vi "Keyence.Gui.vi"(8 "error in":errorcluster, 11 "Idx":i32) -> (0 "error out":errorcluster)   [LabVIEW 2016]
doc: "The function checks for actual position and move to desired absolute position. Then depending on the settings function can check again for position and make retries with lower speed.\n\n#retries - the number of retries to move the motor exactly to position; each time new move is done the speed is divided by 4 (but the min speed is 1) in order to move precisely to positon. possible values are:\n-1: only movement is done without checking whether position was reached\n0: one movemnt is done and then checking whether position was reached\n1: the max number of retries after one unsuccessful movents; with each new movment speed is decreased by 4 and new check is done; if the posiition is in given range function is done\n\nrange[mm] - the max range when checking for the position in range; the minimal value is 0.01mm; the position status is returned as \"Status\" flags"
uses:
  Keyence.BankGui1.ctl
  Keyence.BankGui2.ctl
  Keyence.Data.Status.State.ctl
  Station/Station.State.ctl
  tools/Translator/Translator.Message.ctl
  tools/Translator/Translator.FormatMessage.vi
  Global/ApplicationGlobal.vi
  tools/Config/Config.Global.vi
  Keyence.Global.vi
  Station/Station.Global.vi
  tools/Translator/Translator.Global.vi
panel:
  in  "AutoTune":bool
  in  "Bank2":T1 caption="Bank"
  out "Status":string caption="Code 2"
  out "CodeLevel":string
  out "CodeClass":string
  out "Code":string
  in  "ExitButton":bool
  out "Hider":bool
  in  "ResetPeriod":i32 caption="Reset [s]"
  in  "ReconenctPeriod":i32 caption="Reconect [s]"
  in  "Bank":T2
  in  "Timeout [ms]":i32=1000
  in  "Retries":i32
  in  "IP":string="192.168.0.10"
  out "Image":picture
  out "Hider2":bool
  in  "ScanButton":bool
  in  "TuneButton":bool
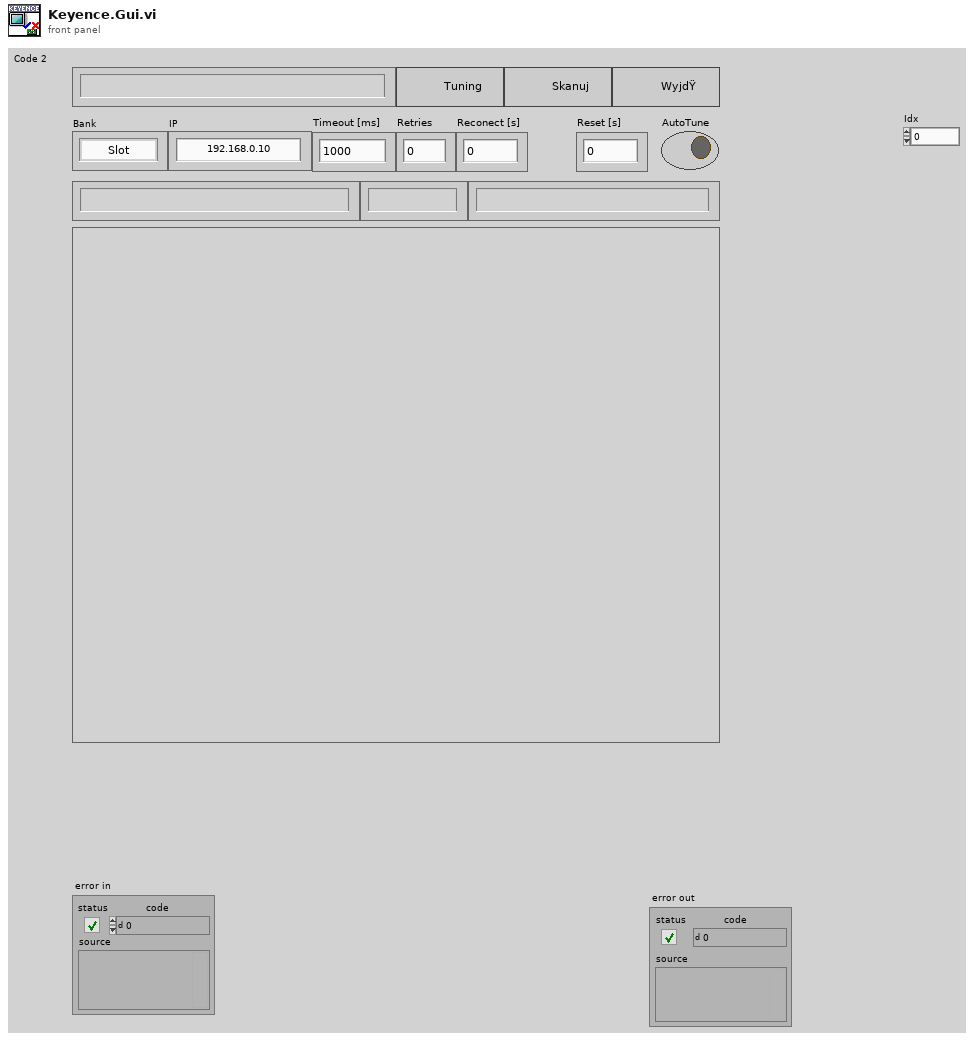
[diagram p1: front panel]
types:
  T1 = typedef "Keyence.BankGui2.ctl" = enum8{"WabcoProd", "WabcoPlate", "ClientProd", "ClientPlate", "TotalQuant", "SerialNo"}
  T2 = typedef "Keyence.BankGui1.ctl" = enum8{"Slot", "A-1", "B-1", "A-2", "B-2"}
  T3 = enum8{"Enabled", "Disabled", "Disabled and Grayed Out"}
  T4 = typedef "Station.State.ctl" = enum16{"Idle", "Ready", "Run", "Stop", "Error", "Home", "Done", "Emg"}
  T5 = typedef "Keyence.Data.Status.State.ctl" = enum16{"First", "Init", "Reset", "Idle", "Scan", "Tune"}
  T6 = typedef "Translator.Message.ctl" = enum16{"-", "Event confirmed", "Log out", "Log in", "Shutdown", "Cancel", "Start", "Begin time", "End time", "Duration", "Service Mode", "Ignore Results", "Serial Format", "On", "Off", "OK", "NOK", "NOK %s", "Home", "Work", "Close", "Open", "In progress...", "Missing", "Empty", "Hardware failure", "Initial", "Default", "Total", "Out of range", "Free disk space is below 1GB - contact technician", "Error %d >> %s", "Error %d >> %s >> %s", "Msg %d >> %s", "Laser msg %d %s", "Laser cmd error %s %d", "Laser cmd failed %s", "Laser cmd warning %s", "Laser disconnected", "Laser status %s", "Laser already started", "Laser job unkonwn %s", "Laser job missing %s", "Laser job select failure %s", "Unable to start laser printing (%s)", "Unable to stop laser printing (%s)", "Laser marking aborted", "Laser marking timeout", "Unable to reset Laser Interlock (%s)", "Unable to trigger Laser. Laser not ready (%s)", "Laser job '%s' coordinates not configured", "Starting %s", "Quitting %s", "Configured", "Initializing", "Quitting", "Loading", "Loaded %d results", "Loaded %d events", "Running", "Stopped", "Summary", "Laser", "Do you want to continue?", "Do you want to delete the configuration?", "The configuration is being used by an order. Unable to delete!", "Press confirm button", "Station is not based. Do you want to exit?", "Station requires changeover. Do you want to run the test?", "Test options are not set as default. Do you want to continue?", "Formatting of WabcoNo is disabled. Do you want to continue?", "Product not detected. Do you want to continue?", "Product scan failed. Do you want to continue?", "Calibration", "Log out?", "System", "All", "IDLE", "Translating...%s", "Not found", "Alarm %s", "Run", "Skip", "Abort", "Repeat", "Please wait...", "Database disconnected", "Database disconnected - changeover disabled!", "Login to database successful", "Login to database failed: %d; %s", "Unable to check the product status of reference %d - database disconnected", "Unable to set the product status of reference %d - database disconnected", "Variant file backup %s", "Read variant (%s)", "Result", "Station armed!", "Station requires changeover!", "Select reference number...", "EMERGENCY BUTTON - press Control button", "EMERGENCY DOOR - press Control button", "Resetting Emergency...", "Unable to reset safety circuit - Emergency Button pressed", "Unable to reset safety circuit - Emergency Side Door open", "Station not based", "Station based", "Station not empty", "Station basing...", "No order", "Press Start to begin new order", "Scanning new order", "Order NOK. Correct or scan again", "Order OK. Press Accept", "Order ready", "Revolver incorrect", "Fork incorrect", "Revolver missing", "Revolver empty", "Container missing", "Offline results", "Offline statistics", "Updating statistics %.1f %%", "DMC Configurator", "Door open", "Close the front door", "Press start button", "Done. Open the front door", "Running...", "Running...%.1f %%", "Pause %s", "Pause %s. NOK container missing", "Pause %s. OK container missing", "Pause %s. Revolver empty", "Pause %s. Revolver missing", "Pause %s. Revolver incorrect", "Pause %s. Fork missing", "Pause %s. Fork incorrect", "Pause %s. Too many failures", "Pause %s. Unloading failure", "Pause %s. One slot is not working", "Pause %s. Part order is done. Empty OK container", "Pause %s. Unable to move product to slot", "Pause %s. Unable to move back product pusher", "Pause %s. Unable to lift product", "Pause %s. Unable to move back product lifter", "Pause %s. Unable to move product arm to Work", "Pause %s. Unable to move product arm to NOK", "Pause %s. Unable to move product arm to OK", "Pause %s. Unable to unsuck the NOK product", "Pause %s. Unable to drop the NOK product", "Pause %s. Product OK missing", "Pause %s. Unable to unsuck the OK product", "Pause %s. Unable to drop the OK product", "Stopping...", "File '%s' is missing", "File '%s' is broken", "File '%s' is running", "Log file started (%s)", "Log file ended (%s)", "Log file stopped (%s)", "Log file ignored (%s)", "Log file exported (%s)", "Log file export failed (%s)", "Wrong serial number in log file", "Wrong reference number in log file", "Test steps are missing", "%s = %.3f", "Process param '%s' not found in DB", "Process param '%s' wrong order", "Process param '%s' value %.3f out of limits (%.3f; %.3f)", "Step%d param '%s' not found in DB", "Step%d param '%s' wrong order", "Step%d param '%s' value %.3f out of limits (%.3f; %.3f)", "Step%d EV '%s' not found in DB", "Step%d EV '%s' wrong order", "\"%s\" not found in DB", "\"%s\" wrong order", "\"%s\" value %.3f out of limits (%.3f; %.3f)", "\"%s\" not found in software", "Process init (%s)", "Process started", "Process restarted", "Process run", "Process done", "Process done - remove OK container", "Process aborted", "Process aborted at work", "Process aborted at home", "Process error", "Process error at home", "Process error at work", "Process close", "Process pause", "Process continue", "Process door open", "Process door close", "Process pause at slot %s due to %s", "Select plate from the order to process", "Do you want to start the process?", "Do you want to continue the process?", "There is unfinished order. Do you want to put the new order?", "Product %s %d OK", "Product %s %d NOK", "Unable to unload the slot %s. Product missing in the slot", "Unable to unload the slot %s. Product already in the arm", "Unable to accept the product as OK. Product missing in slot %s", "Unable to accept the product as OK. Product could not drop into the container at slot %s", "Unable to accept the product as NOK. Product could not drop into the container at slot %s", "Scan failed. Error %s", "Scan failed. Scanner disconnected", "Scan failed. Wrong Wabco number %d, limit (%d,%d)", "Scan failed. Wrong serial number %d, limit (%d,%d)", "Scan failed. Wrong date %d, limit (%d,%d)", "Scan failed. Wrong product wabco number %d (expected %d)", "Scan failed. Wrong product serial number %d (expected > 0)", "Scan OK %s", "Scan failed. Unable to determine table position (%s)", "Scan failed. Timeout", "Tune failed. Scanner disconnected", "Tune failed. Timeout", "%s = %d", "%s = %d->%d", "Unable to set %s = %.2f - Air Pressure Inside off", "Unable to set digital output '%s' = %d", "Unable to activate air pressure inside - timeout", "Unable to activate air pressure inside - aborted", "Unable to switch on Air Main Valve - Air Pressure Inlet off", "Unable to switch on Air Main Valve - Door open", "Unable to switch off Air Main Valve - timeout", "Unable to switch off Air Main Valve - aborted", "Unable to rotate Table - timeout", "Unable to rotate Table - aborted", "Unable to rotate Table - Product Move not in Home position", "Unable to rotate Table - Air Pressure Inside off", "Unable to rotate Table - Product Lift A not in Home position", "Unable to rotate Table - Product Lift B not in Home position", "Unable to rotate Table - unlock before movement timeout", "Unable to rotate Table - lock after movement timeout", "Unable to move Table Lock to %s position - timeout", "Unable to move Table Lock to %s position - aborted", "Unable to move Table Lock to %s position - Air Pressure Inside off", "Unable to move Table Lock to %s position - Table not in position", "Unable to move Product Lift A to %s position - timeout", "Unable to move Product Lift B to %s position - timeout", "Unable to move Product Lift A to %s position - aborted", "Unable to move Product Lift B to %s position - aborted", "Unable to move Product Lift A to %s position - Air Pressure Inside off", "Unable to move Product Lift B to %s position - Air Pressure Inside off", "Unable to move Product Lift A to %s position - Table not locked", "Unable to move Product Lift B to %s position - Table not locked", "Unable to move Product Lift A to %s position - Product Arm not in Work position", "Unable to move Product Lift B to %s position - Product Arm not in Work position", "Unable to set Product Suction Gripper %s to %s - timeout", "Unable to set Product Suction Gripper %s to %s - aborted", "Unable to set Product Suction Gripper %s to %s - Air Pressure Inside off", "Unable to set Product Suction Gripper %s to %s - Table slot unkown", "Unable to move Product Arm to %s position - timeout", "Unable to move Product Arm to %s position - aborted", "Unable to move Product Arm to %s position - Air Pressure Inside off", "Unable to move Product Arm to %s position - Product Lift A not in Home position", "Unable to move Product Arm to %s position - Product Lift B not in Home position", "Unable to move Product to %s position - timeout", "Unable to move Product to %s position - aborted", "Unable to move Product to %s position - Air Pressure Inside off", "Unable to move Product to %s position - Table not in position"}
  T7 = typedef "Keyence.Data.Status.ctl" = cluster{"State":T5, "Ref":refnum<k5>, "Bank":u8, "Version":string, "Model":string, "EndTS":timestamp, "ImgPath":path, "Tuned":bool}
  T8 = typedef "Keyence.CodeDetails.ctl" = cluster{"text":string, "status":bool, "corners":cluster{"X":i32, "Y":i32}[], "level":u8, "class":string, "path":path}
  T9 = typedef "Keyence.Data.Sets.ctl" = cluster{"IP":string, "Timeout_ms":i32, "Retries":i32, "ReconnectPeriod_s":i32, "ResetPeriod_s":i32, "ReadImg":bool}
  T10 = typedef "imagedata.ctl" = cluster{"image type":i32, "image depth":i32, "image":u8[], "mask":u8[], "colors":u32[], "Rectangle":cluster{"left":i16, "top":i16, "right":i16, "bottom":i16}}
  T11 = typedef "Station.Data.ctl" = cluster{"State":T4, "Seq.State":T12, "Seq.BreakReason":T13, "Seq.BreakSource":T14, "Hw failure":bool, "Unconfirmed":bool, "Station empty":bool, "Home err":bool, "Order done":bool, "DUT present":T15, "EmgState":T16, "Sets":T17, "StatusBits":T20}
  T12 = typedef "Sequence.State.ctl" = enum16{"Init", "Idle", "Home", "Work", "Run", "Pause"}
  T13 = typedef "Sequence.Test.BreakReason.ctl" = enum16{"-", "NOK container", "OK container", "Rev empty", "Rev missing", "Rev wrong", "Fork missing", "Fork wrong", "NOK limit", "Unload failure", "Single slot", "Part done", "Err: Prod move work", "Err: Prod move home", "Err: Prod lift work", "Err: Prod lift home", "Err: Prod Arm Work", "Err: Prod Arm NOK", "Err: Prod Arm OK", "Err: Prod NOK suck", "Err: Prod NOK drop", "Err: Prod OK missing", "Err: Prod OK suck", "Err: Prod OK drop"}
  T14 = typedef "Sequence.Test.BreakSource.ctl" = enum16{"-", "A", "B", "A/B"}
  T15 = typedef "FestoCPX.Station.ProdPresent.ctl" = cluster{"Slot1":cluster{"A":bool, "B":bool}, "Slot2":cluster{"A":bool, "B":bool}, "Slot3":cluster{"A":bool, "B":bool}, "Slot4":cluster{"A":bool, "B":bool}, "Final":cluster{"A":bool, "B":bool}, "OK":cluster{"A":bool, "B":bool}, "Container":cluster{"OK":bool, "NOK":bool}}
  T16 = typedef "FestoCPX.Station.EmgState.ctl" = cluster{"Button":bool, "SideDoor":bool, "FrontDoor":bool, "DoorSecured":bool}
  T17 = typedef "Sequence.UserData.ctl" = cluster{"GuiMode":T18, "Test":T19, "ContinueOrder":bool}
  T18 = typedef "Sequence.MainMode.ctl" = enum16{"Process", "Base", "Order", "Manual", "Logs", "Results", "Stats", "DMC Config"}
  T19 = typedef "MainGui.TestOptions.ctl" = cluster{"IgnoreResults":bool, "IgnoreImages":bool, "ServiceMode":bool}
  T20 = typedef "Station.Home.Status.Bits.ctl" = cluster{"Door Close":bool, "Rev OK":bool, "Fork OK":bool, "Container OK":bool, "Station empty":bool}
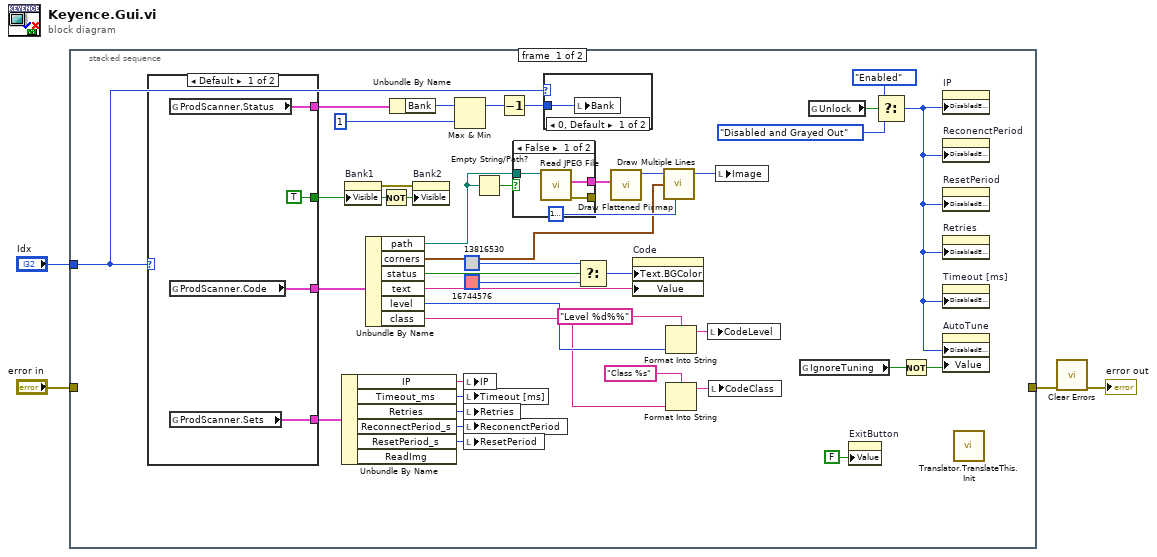
[diagram p0: block diagram]
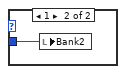
[diagram p2: hidden frame]
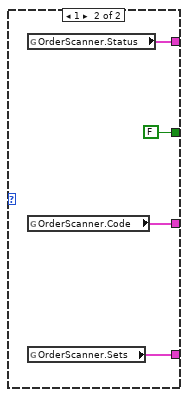
[diagram p3: hidden frame]
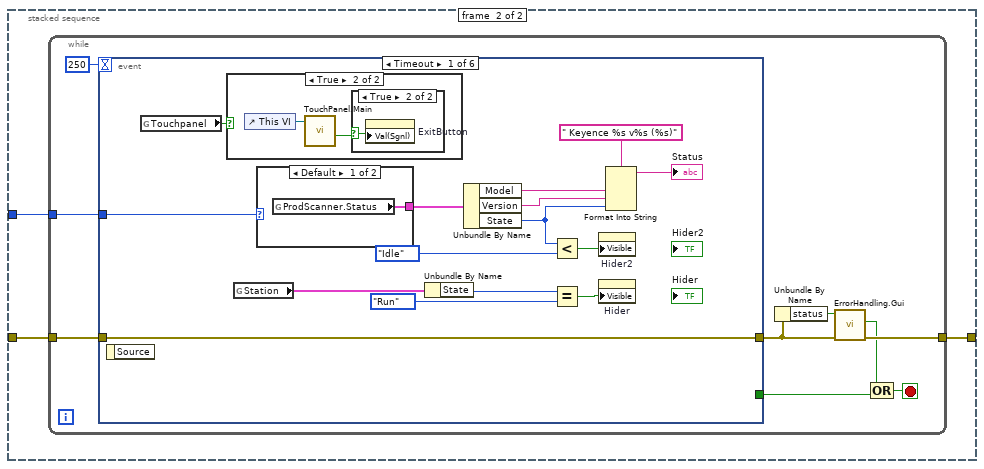
[diagram p5: hidden frame]
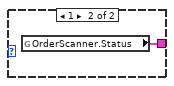
[diagram p6: hidden frame]
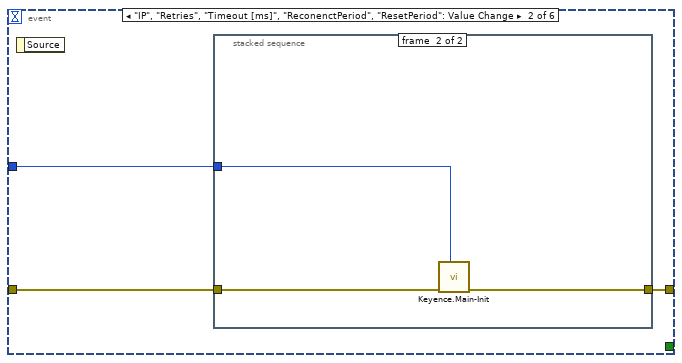
[diagram p9: hidden frame]
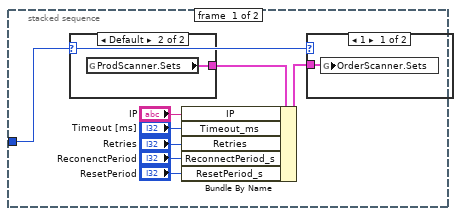
[diagram p10: hidden frame]
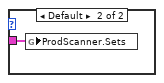
[diagram p11: hidden frame]
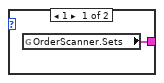
[diagram p12: hidden frame]
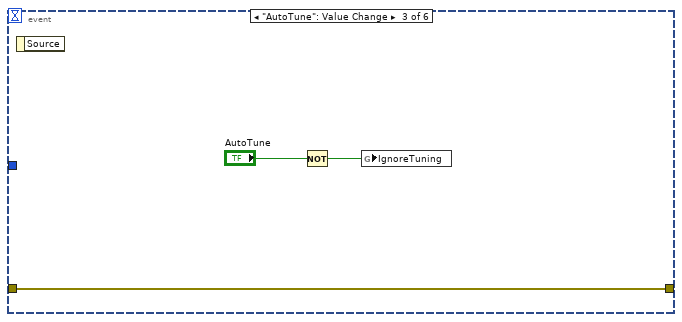
[diagram p13: hidden frame]
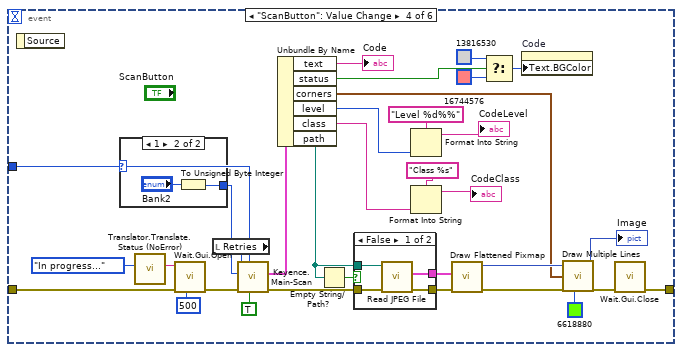
[diagram p14: hidden frame]
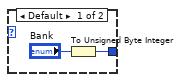
[diagram p15: hidden frame]
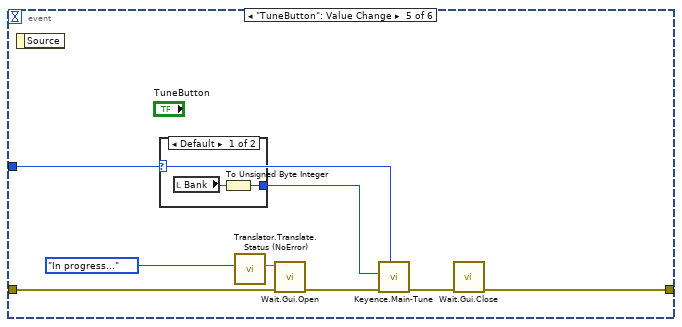
[diagram p17: hidden frame]
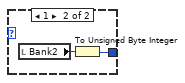
[diagram p18: hidden frame]
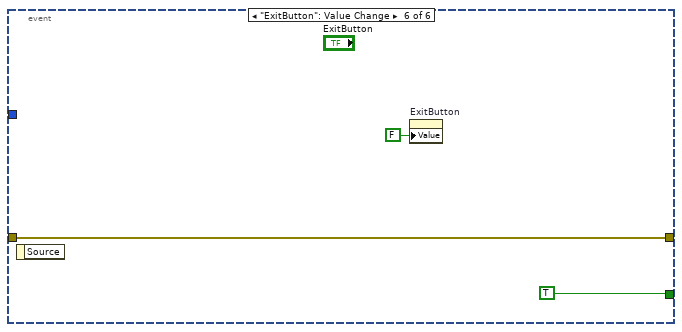
[diagram p19: hidden frame]
diagram:
  n1 = stacked-sequence {
    tunnel: "error in" -> [_ w61]
    tunnel: [_ w60] -> w3
    tunnel: "Idx" -> [w13 w59]
    frame #0 {
      n2 = case shown="Default" w13 {
        tunnel: [w51 w55] -> w30
        tunnel: [w50 w54] -> w24
        tunnel: [w49 w53] -> w21
        tunnel: [TRUE FALSE] -> w15
        frame Default {
          n3 = global read "Keyence.Global.vi" "ProdScanner.Status"() -> (w49:T7)
          n4 = global read "Keyence.Global.vi" "ProdScanner.Code"() -> (w50:T8)
          n5 = global read "Keyence.Global.vi" "ProdScanner.Sets"() -> (w51:T9)
        }
        frame 1 {
          n6 = global read "Keyence.Global.vi" "OrderScanner.Status"() -> (w53:T7)
          n7 = global read "Keyence.Global.vi" "OrderScanner.Code"() -> (w54:T8)
          n8 = global read "Keyence.Global.vi" "OrderScanner.Sets"() -> (w55:T9)
        }
      }
      n9 = Unbundle By Name(w30) -> ("IP"=w29:string, "Timeout_ms"=w28:i32, "Retries"=w27:i32, "ReconnectPeriod_s"=w26:i32, "ResetPeriod_s"=w25:i32)  [unwired: 1 out]
      n10 = property on="Bank1" class="Enum (strict)"("Visible"=w15) -> (error out=w16:errorcluster)  [unwired: 2 in, 1 out]
      n11 = Unbundle By Name(w24) -> ("path"=w23:path, "corners"=w22:cluster{"X":i32, "Y":i32}[], "status"=w39:bool, "text"=w36:string, "level"=w34:u8, "class"=w33:string)
      n12 = Not(x=w15) -> (.not. x?=w14:bool)
      n13 = Unbundle By Name(w21) -> ("Bank"=w20:u8)
      n14 = property on="Bank2" class="Enum (strict)"(error in=w16, "Visible"=w14) -> ()  [unwired: 1 in, 2 out]
      n15 = Max & Min(x=w20, y=u8 1) -> (max(x,y)=w18:u8)  [unwired: 1 out]
      n16 = local write "IP"(w29) -> ()
      n17 = local write "Timeout [ms]"(w28) -> ()
      n18 = local write "Retries"(w27) -> ()
      n19 = local write "ReconenctPeriod"(w26) -> ()
      n20 = local write "ResetPeriod"(w25) -> ()
      n21 = Empty String/Path?(string/path=w23) -> (empty?=w45:bool)
      n22 = Decrement(x=w18) -> (x-1=w19:u8)
      n23 = case shown="False" w45 {
        tunnel: w23 -> [w58 _]
        tunnel: [w57 _] -> _
        tunnel: [w56 _] -> w44
        frame False {
          n24 = call <vilib>:"Read JPEG File.vi"("path to JPEG file"=w58) -> ("error out"=w57:errorcluster, "image data"=w56:T10)  [unwired: 8 in, 1 out]
        }
        frame True {
        }
      }
      n25 = case shown="0, Default" w13 {
        tunnel: w19 -> [w46 w47]
        frame 0, Default {
          n26 = local write "Bank"(w46) -> ()
        }
        frame 1 {
          n27 = local write "Bank2"(w47) -> ()
        }
      }
      n28 = Select(t=u32 13816530, s=w39, f=u32 16744576) -> (s? t:f=w41:u32)
      n29 = call <vilib>:"Draw Flattened Pixmap.vi"("image data"=w44) -> ("new picture"=w37:picture)  [unwired: 8 in]
      n30 = property on="Code" class="Str"("Text.BGColor"=w41, "Value"=w36) -> ()  [unwired: 2 in, 2 out]
      n31 = call <vilib>:"Draw Multiple Lines.vi"("picture"=w37, "line endpoints"=w22, "color(black)"=u32 16777224) -> ("new picture"=w40:picture)  [unwired: 6 in]
      n32 = Format Into String(format string="Level %d%%", w34) -> (resulting string=w32:string)  [unwired: 2 in, 1 out]
      n33 = Format Into String(format string="Class %s", w33) -> (resulting string=w31:string)  [unwired: 2 in, 1 out]
      n34 = local write "CodeLevel"(w32) -> ()
      n35 = local write "CodeClass"(w31) -> ()
      n36 = local write "Image"(w40) -> ()
      n37 = global read "Config.Global.vi" "IgnoreTuning"() -> (w7:bool)
      n38 = global read "ApplicationGlobal.vi" "Unlock"() -> (w10:bool)
      n39 = property on="ExitButton" class="Bool (strict)"("Value"=FALSE ("ExitButton")) -> ()  [unwired: 2 in, 2 out]
      n40 = Select(t=T3."Enabled" ("Disabled"), s=w10, f=T3."Disabled and Grayed Out") -> (s? t:f=w8:T3)
      n41 = Not(x=w7) -> (.not. x?=w6:bool)
      n42 = property on="IP" class="Str"("DisabledEnum"=w8) -> ()  [unwired: 2 in, 2 out]
      n43 = property on="ReconenctPeriod" class="DigNum (strict)"("DisabledEnum"=w8) -> ()  [unwired: 2 in, 2 out]
      n44 = property on="ResetPeriod" class="DigNum (strict)"("DisabledEnum"=w8) -> ()  [unwired: 2 in, 2 out]
      n45 = property on="Retries" class="DigNum (strict)"("DisabledEnum"=w8) -> ()  [unwired: 2 in, 2 out]
      n46 = property on="Timeout [ms]" class="DigNum (strict)"("DisabledEnum"=w8) -> ()  [unwired: 2 in, 2 out]
      n47 = property on="AutoTune" class="Bool (strict)"("DisabledEnum"=w8, "Value"=w6) -> ()  [unwired: 2 in, 2 out]
      n48 = call "Translator.TranslateThis.Init.vi"() -> ()  [unwired: 11 in, 1 out]
    }
    frame #1 {
      n49 = while {
        tunnel: w61 -> [w62]
        tunnel: [w66] -> w60
        tunnel: w59 -> [w68]
        stop <- w63 stop-if-true
        n50 = event shown="[0] Timeout" {
          selector: _ -> [_ _ _ _ _ _]
          dyn-events: _ -> [_ _ _ _ _ _]
          timeout: 250 -> [_ _ _ _ _ _]
          tunnel: [_ _ _ _ _ TRUE] -> w70
          tunnel: [w85 w91 w111 w114 w152 w165] -> w67
          tunnel: w68 -> [w73 w93 _ w123 w159 _]
          tunnel: w62 -> [w85 w92 w111 w118 w155 w165]
          event Timeout {
            n51 = event-data() -> ()  [unwired: 1 in, 1 out]
            n52 = global read "Config.Global.vi" "Touchpanel"() -> (w84:bool)
            n53 = case shown="True" w84 {
              frame False {
              }
              frame True {
                n54 = control-ref of="This VI"() -> (w89:refnum<vi>)
                n55 = call "TouchPanel.Main.vi"("VI ref"=w89) -> ("Canceled"=w88:bool)  [unwired: 8 in, 2 out]
                n56 = case shown="True" w88 {
                  selector: w88 -> [_ w90]
                  frame False {
                  }
                  frame True {
                    n57 = property on="ExitButton" class="Bool (strict)"("Val(Sgnl)"=w90) -> ()  [unwired: 2 in, 2 out]
                  }
                }
              }
            }
            n58 = global read "Station.Global.vi" "Station"() -> (w77:T11)
            n59 = case shown="Default" w73 {
              tunnel: [w86 w87] -> w83
              frame Default {
                n60 = global read "Keyence.Global.vi" "ProdScanner.Status"() -> (w86:T7)
              }
              frame 1 {
                n61 = global read "Keyence.Global.vi" "OrderScanner.Status"() -> (w87:T7)
              }
            }
            n62 = Unbundle By Name(w77) -> ("State"=w76:T4)
            n63 = Unbundle By Name(w83) -> ("Model"=w82:string, "Version"=w74:string, "State"=w79:T5)
            n64 = Less?(x=w79, y=Keyence.Data.Status.State."Idle") -> (x < y?=w71:bool)
            n65 = Equal?(x=w76, y=Station.State."Run") -> (x = y?=w72:bool)
            n66 = property on="Hider2" class="Bool (strict)"("Visible"=w71) -> ()  [unwired: 2 in, 2 out]
            n67 = property on="Hider" class="Bool (strict)"("Visible"=w72) -> ()  [unwired: 2 in, 2 out]
            n68 = Format Into String(format string=" Keyence %s v%s (%s)", w82, w74, w79) -> (resulting string=→"Status":string)  [unwired: 2 in, 1 out]
          }
          event "IP", "Retries", "Timeout [ms]", "ReconenctPeriod", "ResetPeriod": Value Change {
            n69 = event-data() -> ()  [unwired: 1 in, 1 out]
            n70 = stacked-sequence {
              tunnel: w93 -> [w94 w106]
              tunnel: w92 -> [_ w108]
              tunnel: [_ w107] -> w91
              frame #0 {
                n71 = case shown="Default" w94 {
                  tunnel: [w104 w105] -> w101
                  frame 1 {
                    n72 = global read "Keyence.Global.vi" "OrderScanner.Sets"() -> (w104:T9)
                  }
                  frame Default {
                    n73 = global read "Keyence.Global.vi" "ProdScanner.Sets"() -> (w105:T9)
                  }
                }
                n74 = Bundle By Name(cluster=w101, "IP"="IP", "Timeout_ms"="Timeout [ms]", "Retries"="Retries", "ReconnectPeriod_s"="ReconenctPeriod", "ResetPeriod_s"="ResetPeriod") -> (w95:T9)
                n75 = case shown="1" w94 {
                  tunnel: w95 -> [w102 w103]
                  frame 1 {
                    n76 = global write "Keyence.Global.vi" "OrderScanner.Sets"(w102) -> ()
                  }
                  frame Default {
                    n77 = global write "Keyence.Global.vi" "ProdScanner.Sets"(w103) -> ()
                  }
                }
              }
              frame #1 {
                n78 = call "Keyence.Main-Init.vi"("Idx"=w106, "error in"=w108) -> ("error out"=w107:errorcluster)  [unwired: 9 in]
              }
            }
          }
          event "AutoTune": Value Change {
            n79 = event-data() -> ()  [unwired: 1 in, 1 out]
            n80 = Not(x="AutoTune") -> (.not. x?=w109:bool)
            n81 = global write "Config.Global.vi" "IgnoreTuning"(w109) -> ()
          }
          event "ScanButton": Value Change {
            n82 = event-data() -> ()  [unwired: 1 in, 1 out]
            n83 = case shown="1" w123 {
              tunnel: [w143 w145] -> w121
              frame Default {
                n84 = To Unsigned Byte Integer(number="Bank") -> (unsigned 8bit integer=w143:u8)
              }
              frame 1 {
                n85 = To Unsigned Byte Integer(number="Bank2") -> (unsigned 8bit integer=w145:u8)
              }
            }
            n86 = call "Translator.Translate.Status (NoError).vi"("msg"=Translator.Message."In progress...") -> ("Translated Msg"=w116:string)  [unwired: 10 in]
            n87 = call "Wait.Gui.Open.vi"("Delay at open [ms]"=u32 500, "error in (no error)"=w118, "Msg"=w116) -> ("error out"=w117:errorcluster)  [unwired: 8 in]
            n88 = local read "Retries"() -> (w122:i32)
            n89 = call "Keyence.Main-Scan.vi"("get img (F)"=TRUE, "Idx"=w123, "error in"=w117, "Bank"=w121, "Retries (-1: Default)"=w122) -> ("error out"=w142:errorcluster, "Code"=w131:T8)  [unwired: 4 in, 1 out]
            n90 = Unbundle By Name(w131) -> ("text"=→"Code":string, "status"=w133:bool, "corners"=w132:cluster{"X":i32, "Y":i32}[], "level"=w129:u8, "class"=w127:string, "path"=w124:path)
            n91 = Empty String/Path?(string/path=w124) -> (empty?=w141:bool)
            n92 = case shown="False" w141 {
              tunnel: w142 -> [w150 w151]
              tunnel: w124 -> [w149 _]
              tunnel: [w148 w151] -> w115
              tunnel: [w147 _] -> w140
              frame False {
                n93 = call <vilib>:"Read JPEG File.vi"("error in (no error)"=w150, "path to JPEG file"=w149) -> ("error out"=w148:errorcluster, "image data"=w147:T10)  [unwired: 7 in, 1 out]
              }
              frame True {
              }
            }
            n94 = Format Into String(format string="Level %d%%", w129) -> (resulting string=→"CodeLevel":string)  [unwired: 2 in, 1 out]
            n95 = Format Into String(format string="Class %s", w127) -> (resulting string=→"CodeClass":string)  [unwired: 2 in, 1 out]
            n96 = call <vilib>:"Draw Flattened Pixmap.vi"("image data"=w140) -> ("new picture"=w136:picture)  [unwired: 8 in]
            n97 = Select(t=u32 13816530, s=w133, f=u32 16744576) -> (s? t:f=w137:u32)
            n98 = property on="Code" class="Str"("Text.BGColor"=w137) -> ()  [unwired: 2 in, 2 out]
            n99 = call <vilib>:"Draw Multiple Lines.vi"("picture"=w136, "line endpoints"=w132, "color(black)"=u32 6618880) -> ("new picture"=→"Image":picture)  [unwired: 6 in]
            n100 = call "Wait.Gui.Close.vi"("error in (no error)"=w115) -> ("error out"=w114:errorcluster)  [unwired: 10 in]
          }
          event "TuneButton": Value Change {
            n101 = event-data() -> ()  [unwired: 1 in, 1 out]
            n102 = case shown="Default" w159 {
              tunnel: [w161 w163] -> w158
              frame Default {
                n103 = local read "Bank"() -> (w160:T2)
                n104 = To Unsigned Byte Integer(number=w160) -> (unsigned 8bit integer=w161:u8)
              }
              frame 1 {
                n105 = local read "Bank2"() -> (w162:T1)
                n106 = To Unsigned Byte Integer(number=w162) -> (unsigned 8bit integer=w163:u8)
              }
            }
            n107 = call "Translator.Translate.Status (NoError).vi"("msg"=Translator.Message."In progress...") -> ("Translated Msg"=w156:string)  [unwired: 10 in]
            n108 = call "Wait.Gui.Open.vi"("error in (no error)"=w155, "Msg"=w156) -> ("error out"=w154:errorcluster)  [unwired: 9 in]
            n109 = call "Keyence.Main-Tune.vi"("Idx"=w159, "error in"=w154, "Bank"=w158) -> ("error out"=w153:errorcluster)  [unwired: 5 in, 3 out]
            n110 = call "Wait.Gui.Close.vi"("error in (no error)"=w153) -> ("error out"=w152:errorcluster)  [unwired: 10 in]
          }
          event "ExitButton": Value Change {
            n111 = event-data() -> ()  [unwired: 1 in, 1 out]
            n112 = property on="ExitButton" class="Bool (strict)"("Value"=FALSE ("ExitButton")) -> ()  [unwired: 2 in, 2 out]
          }
        }
        n113 = Unbundle By Name(w67) -> ("status"=w65:bool)
        n114 = call "ErrorHandling.Gui.vi"("error in (no error)"=w67, "~Show? (T)"=w65) -> ("error out"=w66:errorcluster, "~close?"=w64:bool)  [unwired: 8 in]
        n115 = Compound Arithmetic op=OR(w64, w70) -> (w63:bool)
      }
    }
  }
  n116 = call <vilib>:"Clear Errors.vi"("error in (no error)"=w3) -> ("error out"=→"error out":errorcluster)  [unwired: 5 in, 1 out]
